vi "MS Multiswitch.vi"() -> ()   [LabVIEW 2012]
uses:
  Type Defs/4 Way Button.ctl
panel:
  out "Mode Select":enum8{"Off", "Stby", "Hold", "Run"}(ring)
  in  "OldVal":T1
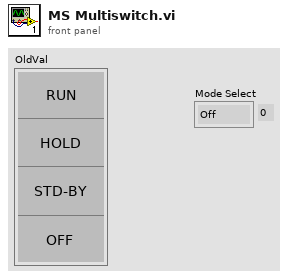
[diagram p1: front panel]
types:
  T1 = typedef "4 Way Button.ctl" = cluster{"Off":bool, "Standby":bool, "Hold":bool, "Run":bool}
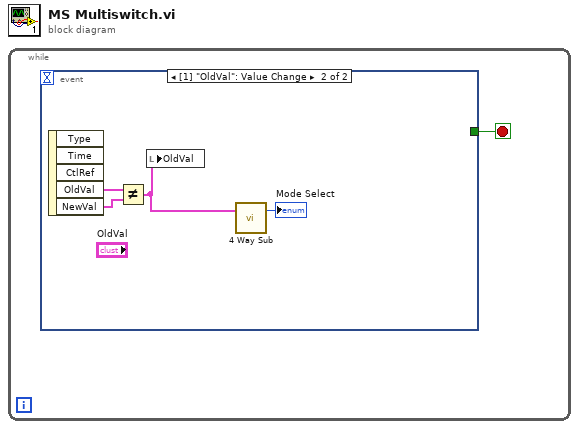
[diagram p0: block diagram]
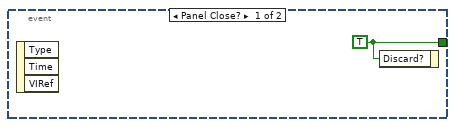
[diagram p2: hidden frame]
diagram:
  n1 = while {
    stop <- w1 stop-if-true
    n2 = event shown="[1] \"OldVal\": Value Change" {
      selector: _ -> [_ _]
      dyn-events: _ -> [_ _]
      timeout: _ -> [_ _]
      tunnel: [w2 _] -> w1
      event Panel Close? {
        w2 = TRUE
        n3 = event-data() -> ()  [unwired: 1 in, 3 out]
        n4 = event-data("Discard?"=w2) -> ()  [unwired: 1 in, 1 out]
      }
      event Value Change {
        n5 = event-data() -> ("OldVal"=w6:T1, "NewVal"=w5:T1)  [unwired: 1 in, 3 out]
        n6 = Not Equal?(x=w6, y=w5) -> (x != y?=w4:T1)
        n7 = local write "OldVal"(w4) -> ()
        n8 = call "4 Way Sub.vi"("OldVal"=w4) -> ("Mode Select"=→"Mode Select":enum8{"Off", "Stby", "Hold", "Run"})  [unwired: 2 in]
      }
    }
  }
